vi "serial_command.vi"(0 "VISA in":refnum<visa-resource-name>, 2 "start byte":string="Ý", 5 "operation enum":T1, 7 "command code enum":T2, 9 "data":string="\u0001\u0010h\r¬\r¬\u0000d\u0000d\tÄ\u0006Ö", 11 "error in":errorcluster, 13 "stop byte":string="w") -> (1 "length":u8, 3 "checksum":u16, 4 "VISA out":refnum<visa-resource-name>, 6 "data":string, 8 "error":string, 12 "assembled command":string, 14 "disassembled command":string, 15 "error out":errorcluster)   [LabVIEW 2019]
uses:
  typedefs/command.ctl
  typedefs/operation.ctl
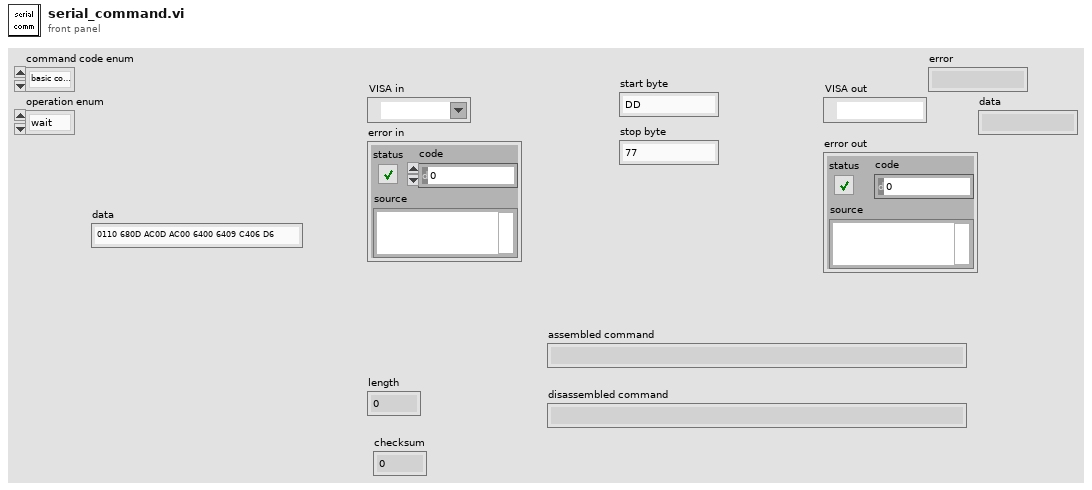
[diagram p1: front panel]
types:
  T1 = typedef "operation.ctl" = enum16{"wait", "read", "write", "action"}
  T2 = typedef "command.ctl" = enum16{"basic configuration", "test configuration", "converter configuration", "reset", "start", "next cell", "next state"}
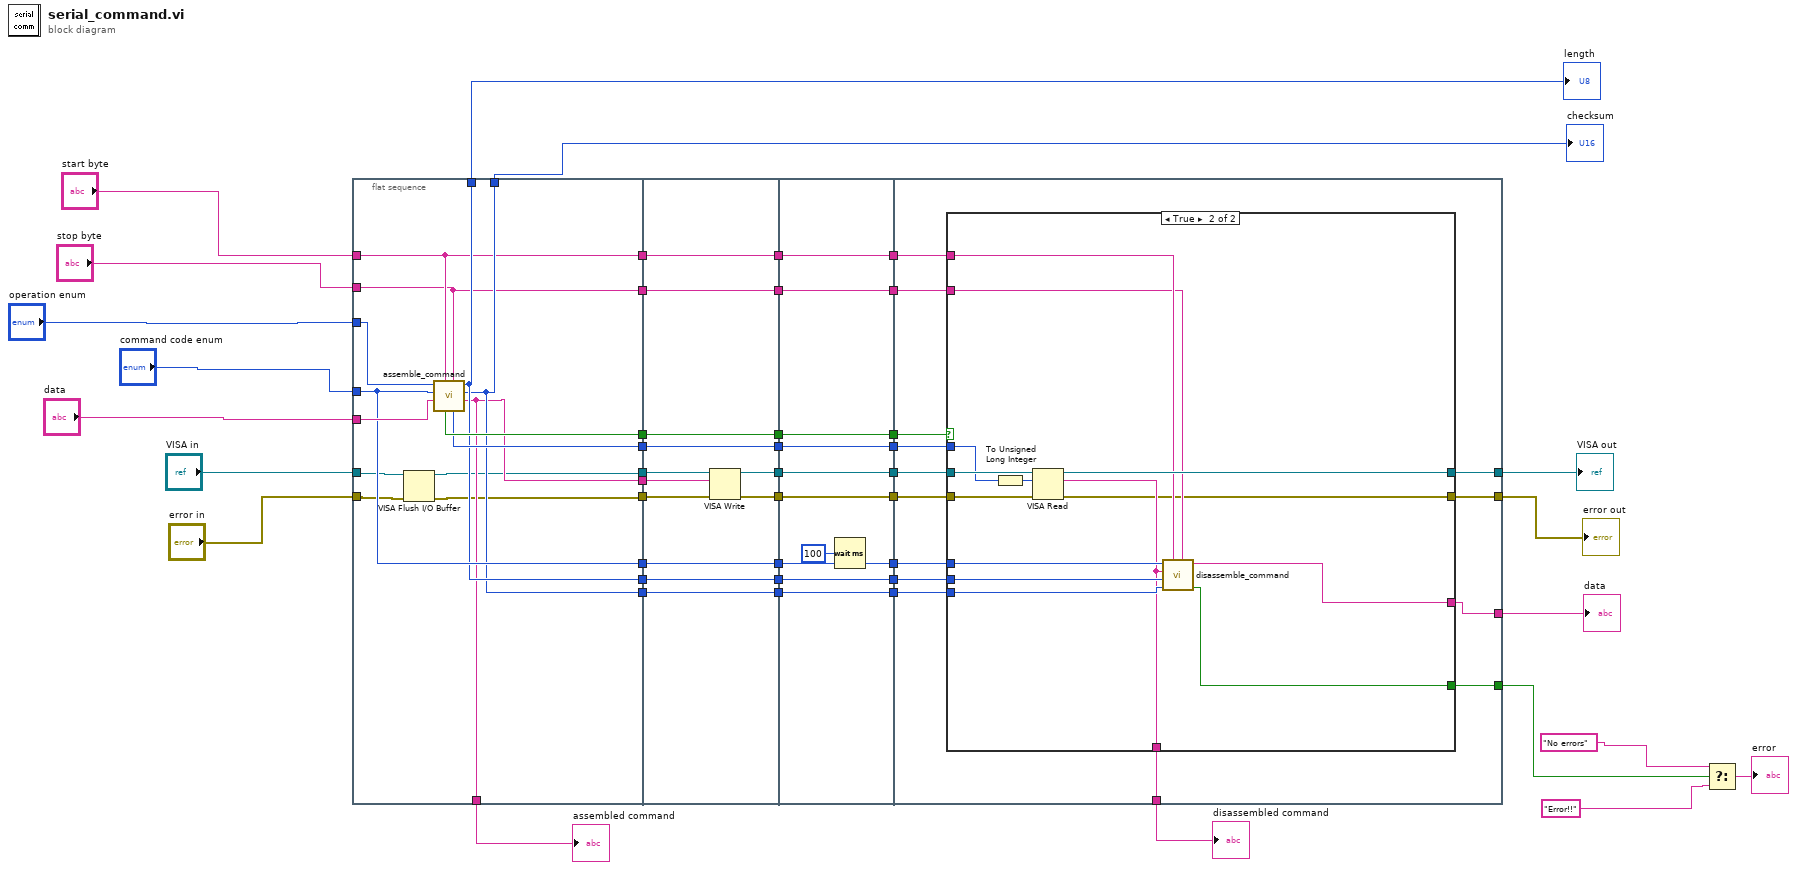
[diagram p0: block diagram]
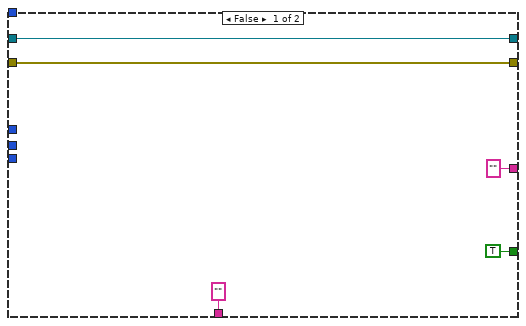
[diagram p2: hidden frame]
diagram:
  n1 = flat-sequence {
    tunnel: "operation enum" -> [w60]
    tunnel: "command code enum" -> [w56]
    tunnel: "data" -> [w59]
    tunnel: "VISA in" -> [w50]
    tunnel: [w47] -> w44
    tunnel: [w48] -> w43
    tunnel: "error in" -> [w49]
    tunnel: [w51] -> w41
    tunnel: [w58] -> w40
    tunnel: [w57] -> w33
    tunnel: [w56] -> w28
    tunnel: [w55] -> w25
    tunnel: [w54] -> w22
    tunnel: [w55] -> w19
    tunnel: [w54] -> w18
    tunnel: "start byte" -> [w53]
    tunnel: "stop byte" -> [w52]
    tunnel: [w53] -> w13
    tunnel: [w52] -> w10
    tunnel: [w51] -> w9
    tunnel: w44 -> [w72]
    tunnel: w43 -> [w71]
    tunnel: w41 -> [w70]
    tunnel: w40 -> [w69]
    tunnel: [w69] -> w39
    tunnel: [w68] -> w37
    tunnel: [w67] -> w35
    tunnel: w33 -> [w66]
    tunnel: [w66] -> w32
    tunnel: w28 -> [w65]
    tunnel: [w65] -> w27
    tunnel: w25 -> [w64]
    tunnel: [w64] -> w24
    tunnel: w22 -> [w63]
    tunnel: [w63] -> w21
    tunnel: [w62] -> w14
    tunnel: w13 -> [w62]
    tunnel: [w61] -> w11
    tunnel: w10 -> [w61]
    tunnel: w39 -> [w81]
    tunnel: [w81] -> w38
    tunnel: w37 -> [w80]
    tunnel: [w80] -> w36
    tunnel: w35 -> [w79]
    tunnel: [w79] -> w34
    tunnel: w32 -> [w78]
    tunnel: [w78] -> w31
    tunnel: w27 -> [w77]
    tunnel: [w77] -> w26
    tunnel: w24 -> [w76]
    tunnel: [w76] -> w23
    tunnel: w21 -> [w75]
    tunnel: [w75] -> w20
    tunnel: [w74] -> w15
    tunnel: w14 -> [w74]
    tunnel: [w73] -> w12
    tunnel: w11 -> [w73]
    tunnel: w38 -> [w96]
    tunnel: w36 -> [w95]
    tunnel: w34 -> [w94]
    tunnel: w31 -> [w93]
    tunnel: [w92] -> w30
    tunnel: [w91] -> w29
    tunnel: w26 -> [w90]
    tunnel: w23 -> [w89]
    tunnel: w20 -> [w88]
    tunnel: w15 -> [w87]
    tunnel: w12 -> [w86]
    tunnel: [w85] -> w5
    tunnel: [w84] -> w8
    tunnel: [w83] -> w1
    frame #0 {
      n2 = VISA Flush I/O Buffer(VISA resource name=w50, error in (no error)=w49) -> (VISA resource name out=w47:refnum<visa-resource-name>, error out=w48:errorcluster)  [unwired: 1 in]
      n3 = call "assemble_command.vi"("stop byte"=w52, "start byte"=w53, "data"=w59, "command code enum"=w56, "operation enum"=w60) -> ("assembled command"=w51:string, "checksum"=w54:u16, "length"=w55:u8, "size of answer"=w57:u8, "requires an answer?"=w58:bool)  [unwired: 2 in]
    }
    frame #1 {
      n4 = VISA Write(VISA resource name=w72, write buffer=w70, error in (no error)=w71) -> (VISA resource name out=w68:refnum<visa-resource-name>, error out=w67:errorcluster)  [unwired: 1 out]
    }
    frame #2 {
      n5 = Wait (ms)(milliseconds to wait=u32 100) -> ()  [unwired: 1 out]
    }
    frame #3 {
      n6 = case shown="True" w96 {
        tunnel: w95 -> [w101 w115]
        tunnel: w94 -> [w100 w114]
        tunnel: w93 -> [_ w112]
        tunnel: [w101 w111] -> w92
        tunnel: [w100 w103] -> w91
        tunnel: w90 -> [_ w110]
        tunnel: w89 -> [_ w109]
        tunnel: w88 -> [_ w108]
        tunnel: w87 -> [_ w107]
        tunnel: w86 -> [_ w106]
        tunnel: [TRUE ("tests") w105] -> w85
        tunnel: ["" ("read buffer") w104] -> w84
        tunnel: ["" ("data") w102] -> w83
        frame False {
        }
        frame True {
          n7 = To Unsigned Long Integer(number=w112) -> (unsigned 32bit integer=w113:u32)
          n8 = VISA Read(VISA resource name=w115, byte count=w113, error in (no error)=w114) -> (VISA resource name out=w111:refnum<visa-resource-name>, read buffer=w104:string, error out=w103:errorcluster)  [unwired: 1 out]
          n9 = call "disassemble_command.vi"("stop byte"=w106, "start byte"=w107, "expected checksum"=w108, "expected size of data"=w109, "received from serial"=w104, "command code enum"=w110) -> ("tests"=w105:bool, "data"=w102:string)  [unwired: 4 in]
        }
      }
    }
  }
  n10 = Select(t="No errors", s=w5, f="Error!!") -> (s? t:f=→"error":string)
  "VISA out" <- w30
  "error out" <- w29
  "length" <- w19
  "checksum" <- w18
  "assembled command" <- w9
  "disassembled command" <- w8
  "data" <- w1
